vi "High G Data GFV.vi"(1 "Action":T1, 7 "LEIN reply":T2={"Reply msg(cmdif no reply)"={"SID"=0, "ANF"=FALSE, "CMD"=enum."TASK", "DATA"=[]}, "Reply time"=timestamp(0 s since 1904-01-01), "Valid reply"=FALSE}, 11 "error in (no error)":errorcluster, 12 "Max values in each buffer":i32=6000) -> (6 "X axis":dbl[](array[numeric]), 8 "Y axis":dbl[](array[numeric]), 10 "Z axis":dbl[](array[numeric]), 14 "Data added":bool, 15 "error out":errorcluster)   [LabVIEW 2011]
uses:
  LEINmaster/Defenitions/LEIN Reply Holder.ctl
  LEINmaster/Defenitions/LEIN CMD Cluster.ctl
  LEINmaster/Defenitions/LEIN CMD List.ctl
  high G data GFV Action.ctl
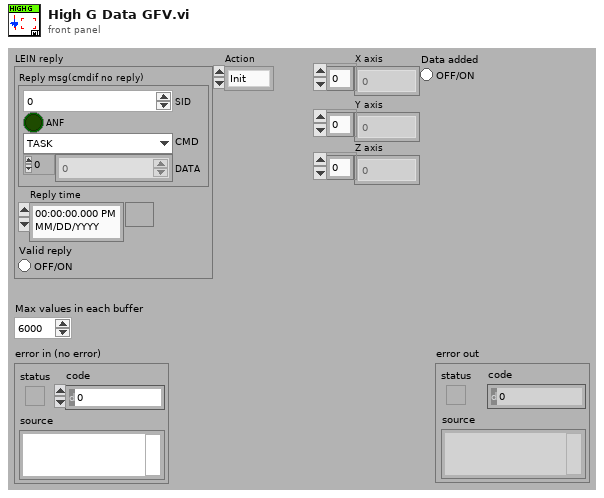
[diagram p1: front panel]
types:
  T1 = typedef "high G data GFV Action.ctl" = enum16{"Init", "Add data", "Get"}
  T2 = typedef "LEIN Reply Holder.ctl" = cluster{"Reply msg(cmdif no reply)":T3, "Reply time":timestamp, "Valid reply":bool}
  T3 = typedef "LEIN CMD Cluster.ctl" = cluster{"SID":u8, "ANF":bool, "CMD":T4, "DATA":u8[]}
  T4 = typedef "LEIN CMD List.ctl" = enum8{"ACTI", "TASK", "RES0", "STAT", "RES1", "RES2", "RES3", "USER"}
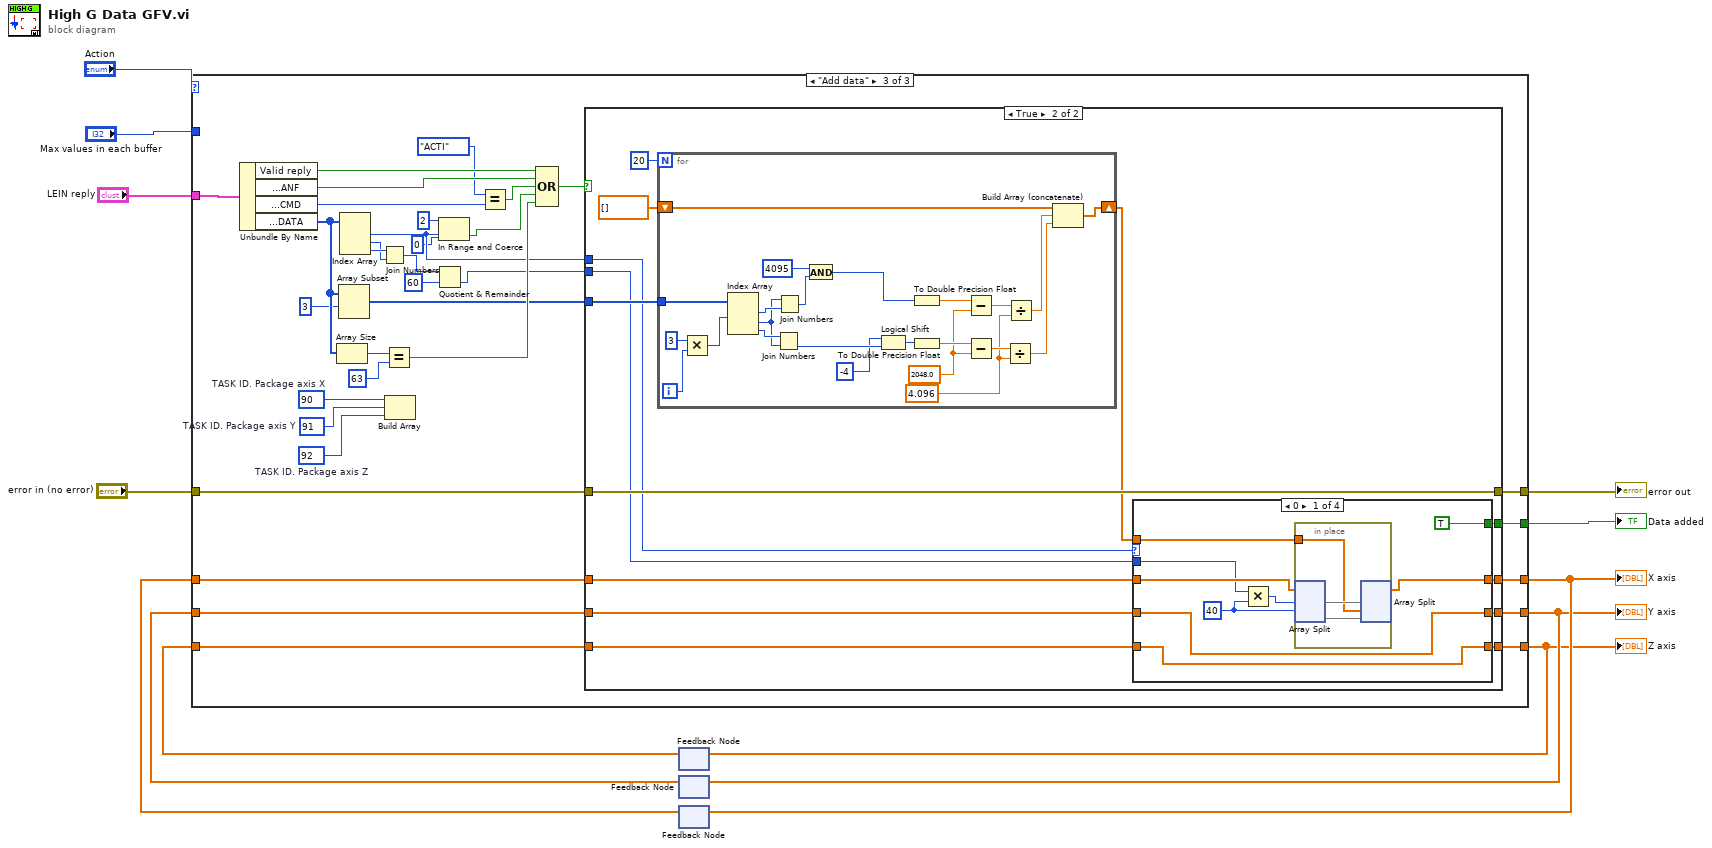
[diagram p0: block diagram]
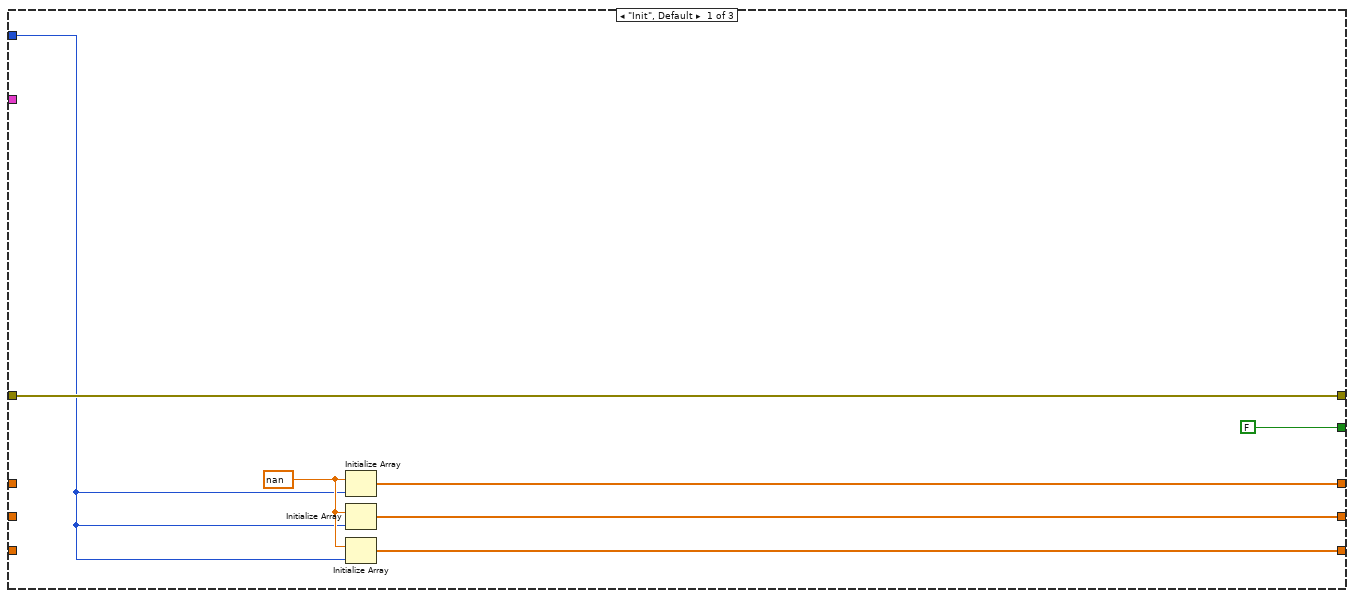
[diagram p2: hidden frame]
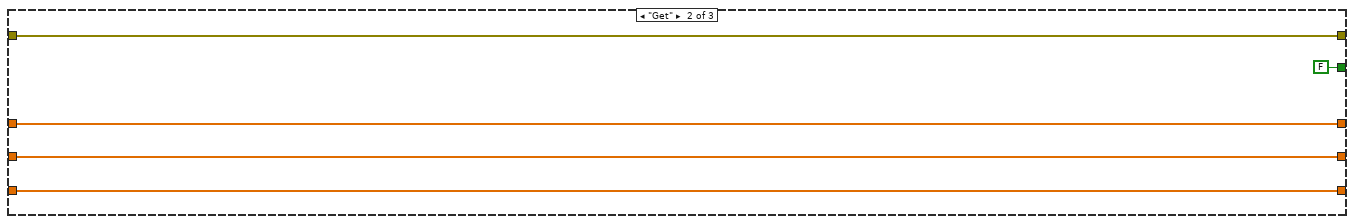
[diagram p3: hidden frame]
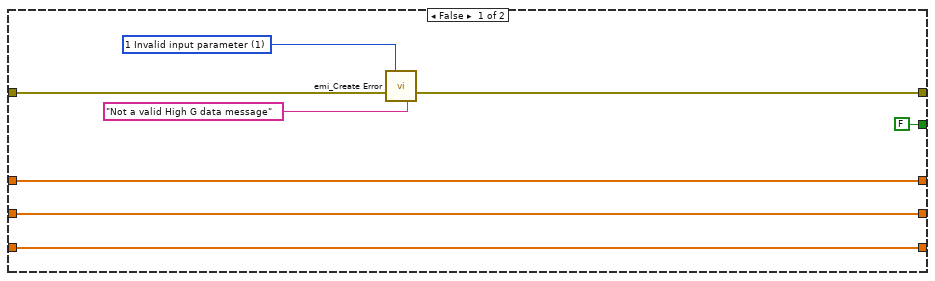
[diagram p4: hidden frame]
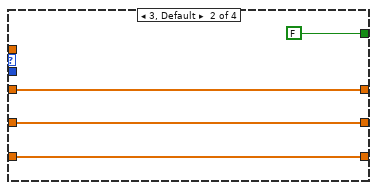
[diagram p5: hidden frame]
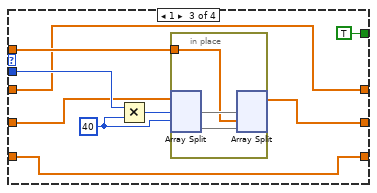
[diagram p6: hidden frame]
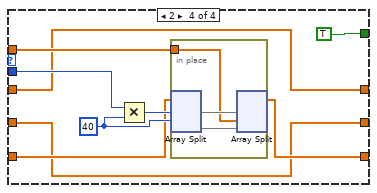
[diagram p7: hidden frame]
diagram:
  n1 = feedback #1() -> (w4:dbl[])  [unwired: 1 in]
  n2 = feedback #2() -> (w5:dbl[])  [unwired: 1 in]
  n3 = feedback #3() -> (w6:dbl[])  [unwired: 1 in]
  n4 = case shown="\"Add data\"" "Action" {
    tunnel: "LEIN reply" -> [_ _ w58]
    tunnel: [w15 w24 w42] -> w9
    tunnel: "error in (no error)" -> [w15 w24 w41]
    tunnel: "Max values in each buffer" -> [w13 _ _]
    tunnel: [w18 w23 w37] -> w7
    tunnel: w6 -> [_ w23 w36]
    tunnel: [w17 w22 w35] -> w3
    tunnel: [w16 w21 w33] -> w2
    tunnel: w5 -> [_ w22 w34]
    tunnel: w4 -> [_ w21 w32]
    tunnel: [FALSE FALSE w31] -> w1
    frame "Init", Default {
      w19 = nan
      n5 = Initialize Array(w19, w13) -> (w18:dbl[])
      n6 = Initialize Array(w19, w13) -> (w17:dbl[])
      n7 = Initialize Array(w19, w13) -> (w16:dbl[])
    }
    frame "Get" {
    }
    frame "Add data" {
      w55 = u8 92  # TASK ID. Package axis Z
      w56 = u8 91  # TASK ID. Package axis Y
      w57 = u8 90  # TASK ID. Package axis X
      n8 = Unbundle By Name(w58) -> ("Valid reply"=w54:bool, "Reply msg(cmdif no reply).ANF"=w53:bool, "Reply msg(cmdif no reply).CMD"=w52:T4, "Reply msg(cmdif no reply).DATA"=w45:u8[])
      n9 = Array Size(array=w45) -> (size(s)=w49:i32)
      n10 = Array Subset(array=w45, index=3) -> (w39:u8[])  [unwired: 1 in]
      n11 = Index Array(array=w45) -> (element #1=w30:u8, element #2=w46:u8, element #3=w47:u8)  [unwired: 3 in]
      n12 = Join Numbers(hi=w47, lo=w46) -> ((hi.lo)=w38:u16)
      n13 = Equal?(x=w49, y=63) -> (x = y?=w48:bool)
      n14 = Build Array(w57, w56, w55) -> ()  [unwired: 1 out]
      n15 = Quotient & Remainder(x=w38, y=u16 60) -> (floor(x/y)=w25:u16)  [unwired: 1 out]
      n16 = In Range and Coerce(upper limit=u8 2, x=w30, lower limit=u8 0) -> (In Range?=w27:bool)  [unwired: 1 out]
      n17 = Equal?(x=LEIN_CMD_List."ACTI", y=w52) -> (x = y?=w50:bool)
      n18 = Compound Arithmetic op=OR(w54, w53, w50, w27, w48) -> (w43:bool)
      n19 = case shown="True" w43 {
        tunnel: [w65 w80] -> w42
        tunnel: w41 -> [w66 w80]
        tunnel: w39 -> [_ w79]
        tunnel: w30 -> [_ w76]
        tunnel: w25 -> [_ w70]
        tunnel: [w62 w75] -> w37
        tunnel: w36 -> [w62 w74]
        tunnel: [w61 w68] -> w35
        tunnel: w34 -> [w61 w73]
        tunnel: [w60 w72] -> w33
        tunnel: w32 -> [w60 w71]
        tunnel: [FALSE w67] -> w31
        frame False {
          w64 = 1 items=["0 No Error"=0, "1 Invalid input parameter"=1, "6 Generic file IO "=6, "7 File not Found"=7, "35 Generic Pring Error"=35, "37 Device not Found"=37, "39 Device Unit Error"=39, "40 Could fot Open Device"=40, "42 Generic Error"=42, "52 Unknown Message"=52, "98 Bad File type"=98, "99 Bad File Version"=99, "100 Bad Data in File"=100, "1018 Unspecefied Error"=1018, "1041 Incorrect Password"=1041, "1043 Feature not in this version"=1043, "1109 Unsuported Data type"=1109, "1444 Did not close sucessfully"=1444] ("Error Code")
          n20 = call "emi_Create Error.vi"("Error Code"=w64, "error in (no error)"=w66, "Append String(\"\")"="Not a valid High G data message" ("Append String(\"\")")) -> ("error out"=w65:errorcluster)  [unwired: 12 in]
        }
        frame True {
          n21 = for {
            N: 20 -> [_]
            tunnel: w79 -> [w136]
            shift-right: [w132] -> w69
            shift-left: dbl[] [] -> [w133]
            i -> [w143]
            w121 = 4.096 ("y")
            w124 = 2048.0 ("y")
            n22 = Multiply(x=3, y=w143) -> (x*y=w135:i32)
            n23 = Index Array(array=w136, index #1=w135) -> (element #1=w141:u8, element #2=w139:u8, element #3=w140:u8)  [unwired: 2 in]
            n24 = Join Numbers(hi=w140, lo=w139) -> ((hi.lo)=w138:u16)
            n25 = Join Numbers(hi=w139, lo=w141) -> ((hi.lo)=w128:u16)
            n26 = And(x=u16 4095, y=w128) -> (x .and. y?=w127:u16)
            n27 = Logical Shift(y=i8 -4, x=w138) -> (x << y=w134:u16)
            n28 = To Double Precision Float(number=w127) -> (double precision float=w131:dbl)
            n29 = To Double Precision Float(number=w134) -> (double precision float=w130:dbl)
            n30 = Subtract(x=w131, y=w124) -> (x-y=w126:dbl)
            n31 = Subtract(x=w130, y=w124) -> (x-y=w125:dbl)
            n32 = Divide(x=w125, y=w121) -> (x/y=w122:dbl)
            n33 = Divide(x=w126, y=w121) -> (x/y=w123:dbl)
            n34 = Build Array (concatenate)(w133, w123, w122) -> (w132:dbl[])
          }
          n35 = case shown="0" w76 {
            tunnel: [w85 w96 w98 w113] -> w75
            tunnel: w74 -> [w89 w96 w98 w113]
            tunnel: w73 -> [w84 w95 w100 w110]
            tunnel: [w83 w94 w102 w111] -> w72
            tunnel: w71 -> [w83 w94 w102 w112]
            tunnel: w70 -> [w86 _ w103 w115]
            tunnel: w69 -> [w82 _ w101 w114]
            tunnel: [w84 w95 w99 w110] -> w68
            tunnel: [TRUE FALSE TRUE TRUE] -> w67
            frame 0 {
              w87 = 40
              n36 = Multiply(x=w86, y=w87) -> (x*y=w88:i32)
              n37 = in-place {
                in-place-border: w82 -> [w90]
                n38 = in-place-split #4(w89, w88, w87) -> (w92:dbl[], w91:dbl[])  [unwired: 1 out]
                n39 = in-place-split #4(w92, w90, w91) -> (w85:dbl[])  [unwired: 2 out]
              }
            }
            frame 3, Default {
            }
            frame 1 {
              w104 = 40
              n40 = Multiply(x=w103, y=w104) -> (x*y=w105:i32)
              n41 = in-place {
                in-place-border: w101 -> [w106]
                n42 = in-place-split #5(w100, w105, w104) -> (w108:dbl[], w107:dbl[])  [unwired: 1 out]
                n43 = in-place-split #5(w108, w106, w107) -> (w99:dbl[])  [unwired: 2 out]
              }
            }
            frame 2 {
              w116 = 40
              n44 = Multiply(x=w115, y=w116) -> (x*y=w117:i32)
              n45 = in-place {
                in-place-border: w114 -> [w118]
                n46 = in-place-split #6(w112, w117, w116) -> (w120:dbl[], w119:dbl[])  [unwired: 1 out]
                n47 = in-place-split #6(w120, w118, w119) -> (w111:dbl[])  [unwired: 2 out]
              }
            }
          }
        }
      }
    }
  }
  "error out" <- w9
  "X axis" <- w7
  "Y axis" <- w3
  "Z axis" <- w2
  "Data added" <- w1
  n48 = feedback-in #1(w2) -> ()
  n49 = feedback-in #2(w3) -> ()
  n50 = feedback-in #3(w7) -> ()
